vi "DelayQueue.vi"(11 "MessageQueues":T1) -> ()   [LabVIEW 2024]
uses:
  MessageQueues.ctl
  <vilib>/httpClient/ClientHandle.ctl
  <vilib>/httpClient/LabVIEWHTTPClient.lvlib
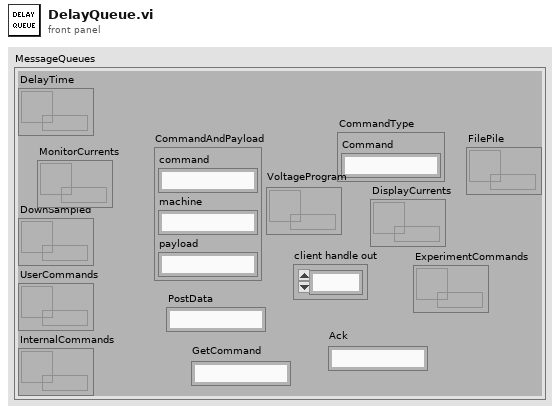
[diagram p1: front panel]
types:
  T1 = typedef "MessageQueues.ctl" = cluster{"DelayTime":refnum<queue>, "DownSampled":refnum<queue>, "UserCommands":refnum<queue>, "InternalCommands":refnum<queue>, "CommandType":cluster{"Command":string}, "CommandAndPayload":cluster{"command":string, "machine":string, "payload":string}, "client handle out":T2, "PostData":string, "GetCommand":string, "Ack":string, "VoltageProgram":refnum<queue>, "ExperimentCommands":refnum<queue>, "DisplayCurrents":refnum<queue>, "MonitorCurrents":refnum<queue>, "FilePile":refnum<queue>}
  T2 = typedef "LabVIEWHTTPClient.lvlib/ClientHandle.ctl" = refnum<k1>
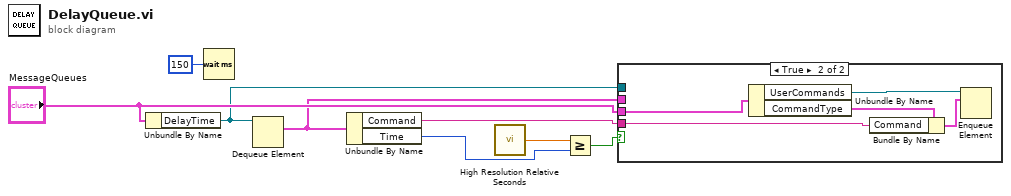
[diagram p0: block diagram]
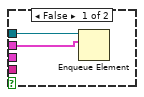
[diagram p2: hidden frame]
diagram:
  n1 = Unbundle By Name("MessageQueues") -> ("DelayTime"=w6:refnum<queue>)
  n2 = Wait (ms)(milliseconds to wait=u32 150) -> ()  [unwired: 1 out]
  n3 = Dequeue Element(queue=w6) -> (element=w1:cluster{"Command":string, "Time":i32})  [unwired: 2 in, 3 out]
  n4 = Unbundle By Name(w1) -> ("Command"=w5:string, "Time"=w2:i32)
  n5 = call <vilib>:"High Resolution Relative Seconds.vi"() -> ("relative seconds"=w3:dbl)
  n6 = Greater Or Equal?(x=w3, y=w2) -> (x >= y?=w4:bool)
  n7 = case shown="True" w4 {
    tunnel: "MessageQueues" -> [_ w13]
    tunnel: w5 -> [_ w15]
    tunnel: w6 -> [w10 _]
    tunnel: w1 -> [w9 _]
    frame False {
      n8 = Enqueue Element(queue=w10, element=w9) -> ()  [unwired: 2 in, 3 out]
    }
    frame True {
      n9 = Unbundle By Name(w13) -> ("UserCommands"=w12:refnum<queue>, "CommandType"=w11:cluster{"Command":string})
      n10 = Bundle By Name(cluster=w11, "Command"=w15) -> (w14:cluster{"Command":string})
      n11 = Enqueue Element(queue=w12, element=w14) -> ()  [unwired: 2 in, 3 out]
    }
  }
